vi "GetDependencyCount.vi"(8 "error in (no error)":errorcluster, 11 "CDependencyInspector in":refnum<class "CDependencyInspection.lvclass">) -> (0 "error out":errorcluster, 1 "Count":i32, 3 "CDependencyInspector out":refnum<class "CDependencyInspection.lvclass">)   [LabVIEW 2020, in "DependencyInspection.lvlib" / "CDependencyInspection.lvclass"]
uses:
  CDependencyInspection.lvclass
  CDependencyInspection.lvclass/CDependencyInspection.ctl
  CDependencyList/CDependencyList.lvclass
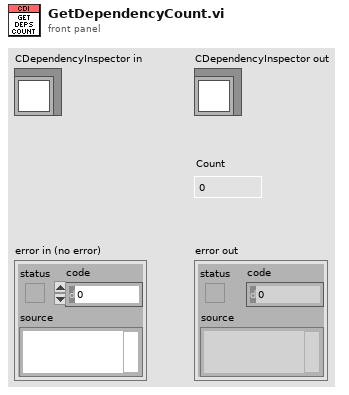
[diagram p1: front panel]
types:
  T1 = typedef "DependencyInspection.lvlib/CDependencyList.lvclass/DependencyList.ctl" = map{string, refnum<class "ILabVIEWItem.lvclass">}
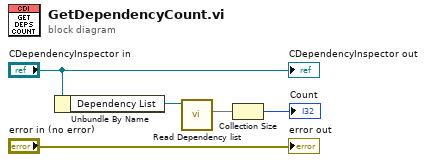
[diagram p0: block diagram]
diagram:
  n1 = Unbundle By Name("CDependencyInspector in") -> ("Dependency List"=w2:refnum<class "CDependencyList.lvclass">)
  n2 = call-dynamic "Read Dependency list.vi"("CDependencyList in"=w2) -> ("Dependency List"=w1:T1)  [unwired: 9 in, 1 out]
  n3 = Collection Size(1:w1) -> (0:→"Count":i32)
  "error out" <- "error in (no error)"
  "CDependencyInspector out" <- "CDependencyInspector in"
